vi "RTI Connext DDS Secure Shapes Reader.vi"() -> ()   [LabVIEW 2012]
doc: "Shows how to subscribe to an existing RTI Connext DDS application: RTI Shapes Demo. It was created using the Tutorial of the Getting Started Guide (<LabVIEW folder>/help/RTI DDS Toolkit for LabVIEW/RTI_DDS_Toolkit_for_LabVIEW_GettingStarted.pdf)."
uses:
  RTI/GIT_HEAD/connextdds/lvdds.1.0/srcLV/lvdds.1.0_package/Examples/ShapesDemo/RTI Connext DDS Shape Type.ctl
  RTI/GIT_HEAD/connextdds/lvdds.1.0/srcLV/lvdds.1.0_package/Types/DDS Sample Info.ctl
  RTI/GIT_HEAD/connextdds/lvdds.1.0/srcLV/lvdds.1.0_package/Types/RTI DDS Advanced Reader Configuration.ctl
  RTI/GIT_HEAD/connextdds/lvdds.1.0/srcLV/lvdds.1.0_package/Types/RTI DDS Security Settings.ctl
  RTI/GIT_HEAD/connextdds/lvdds.1.0/srcLV/lvdds.1.0_package/Types/RTI DDS Basic Security Settings.ctl
  RTI/GIT_HEAD/connextdds/lvdds.1.0/srcLV/lvdds.1.0_package/Types/RTI DDS Advanced Security Settings.ctl
  RTI/GIT_HEAD/connextdds/lvdds.1.0/srcLV/lvdds.1.0_package/Library/LVDDS_library.lvlib
  RTI/GIT_HEAD/connextdds/lvdds.1.0/lib/rtilvdds.dll
panel:
  in  "Domain Id":u32
  in  "Topic Name":string(combo)="Square"
  in  "error in (no error)":errorcluster
  in  "Advanced Reader Configuration":T1
  in  "Enter a shape 'color' to see the square moving in 'XY Graph' and its size in 'shapesize'":string
  out "Sample Info":T2
  out "Return value 2":i32
  out "DDS Data":string[][](table)
  in  "Enable DDS":bool
  in  "ShapeType 2":T3
  out "XY Graph":cluster{"Y":dbl[], "Y":dbl[]}[](graph)
  out "shapesize":i32(slide) scale=0.0..100.0
  in  "Query condition":string
  in  "Stop":bool
  out "Shape 2":T4
  out "Return value":i32
  # "This Example will show Security capabilities using RTI Shapes Demo example. \n\nRTI Shapes Demo is a sample application that demonstrates DDS concepts. It can publish and subscribe to data of type “ShapeType”, which consists of color, x and y coordinates, and a shapesize.  You can use this example to subscribe to Secure Shapes data using  RTI Connext. Run RTI Shapes Demo 5.2.4 or above or the Secure Shapes Writer.vi to publish entities. Start this Shapes Reader example VI, and click on 'DDS  Stopped' below to start reading. Published Shapes data will be displayed. \nIf you want to see one of the shapes moving in the XY Graph, enter its color (in capital letters) in the box below."
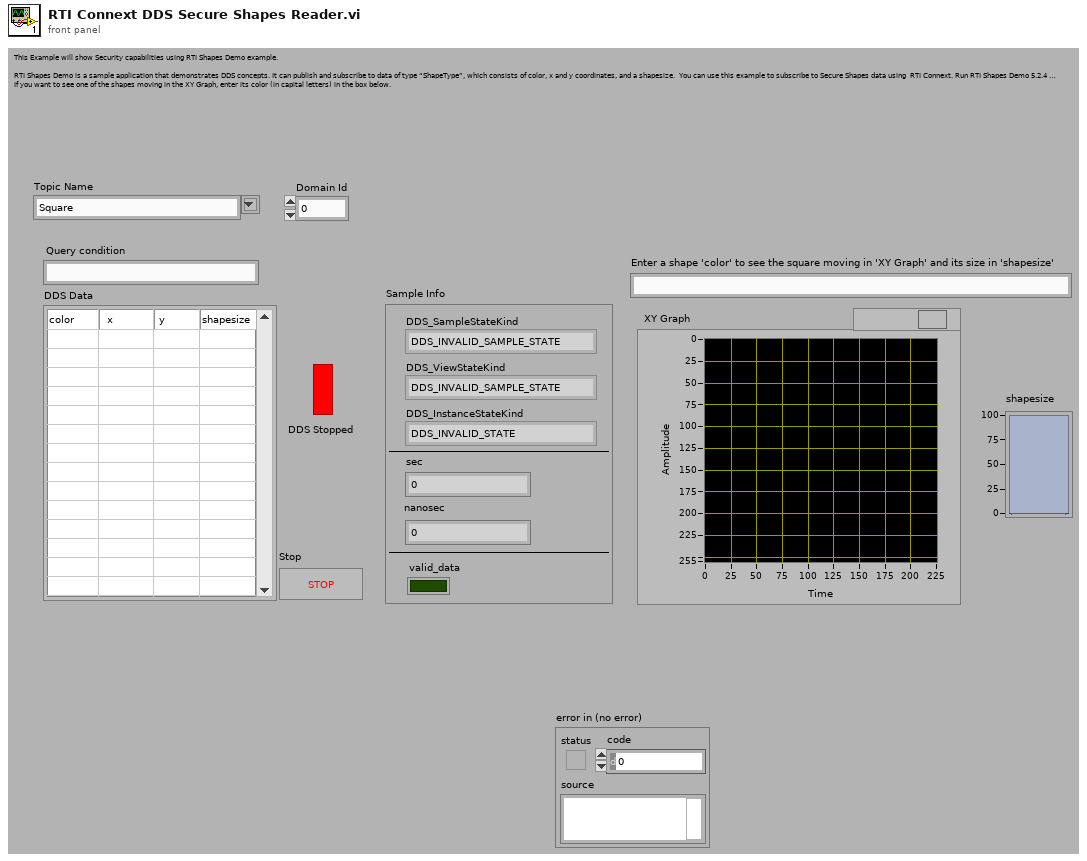
[diagram p1: front panel]
types:
  T1 = typedef "LVDDS_library.lvlib/RTI DDS Advanced Reader Configuration.ctl" = cluster{"typeName":string, "keyName":string, "domainParticipantQoSProfile":string, "dataReaderQoSProfile":string, "forceNewDomainParticipant?":bool, "forceArrayMapping?":bool, "forceExclusiveReader?":bool, "forceRead? (only ExclusiveReader)":bool, "forceUnboundedString?":bool}
  T2 = typedef "LVDDS_library.lvlib/DDS Sample Info.ctl" = cluster{"DDS_SampleStateKind":enum32{"DDS_INVALID_SAMPLE_STATE", "DDS_READ_SAMPLE_STATE", "DDS_NOT_READ_SAMPLE_STATE"}, "DDS_ViewStateKind":enum32{"DDS_INVALID_SAMPLE_STATE", "DDS_NEW_VIEW_STATE", "DDS_NOT_NEW_VIEW_STATE"}, "DDS_InstanceStateKind":enum32{"DDS_INVALID_STATE", "DDS_ALIVE_INSTANCE_STATE", "DDS_NOT_ALIVE_DISPOSED_INSTANCE_STATE", "", "DDS_NOT_ALIVE_NO_WRITERS_INSTANCE_STATE"}, "sec":i32, "nanosec":u32, "valid_data":bool}
  T3 = cluster{"Color":string, "x":i32, "y":i32, "shapesize":i32}
  T4 = typedef "RTI Connext DDS Shape Type.ctl" = cluster{"color":string, "x":i32, "y":i32, "shapesize":i32}
  T5 = typedef "LVDDS_library.lvlib/RTI DDS Security Settings.ctl" = cluster{"Basic Security Settings":T6, "Advanced Security Settings":T7}
  T6 = typedef "LVDDS_library.lvlib/RTI DDS Basic Security Settings.ctl" = cluster{"Identity Certificate Authority (CA)":path, "Identity Certificate (Signed by Identity CA)":path, "Private Key":path, "Permissions Certificate Authority (CA)":path, "Governance Document (Signed by Permissions CA)":path, "Permissions Document (Signed by Permissions CA)":path}
  T7 = typedef "LVDDS_library.lvlib/RTI DDS Advanced Security Settings.ctl" = cluster{"Shared Secret Algorithm":string, "Encryption Algorithm":string, "Certificate Revocation List":path}
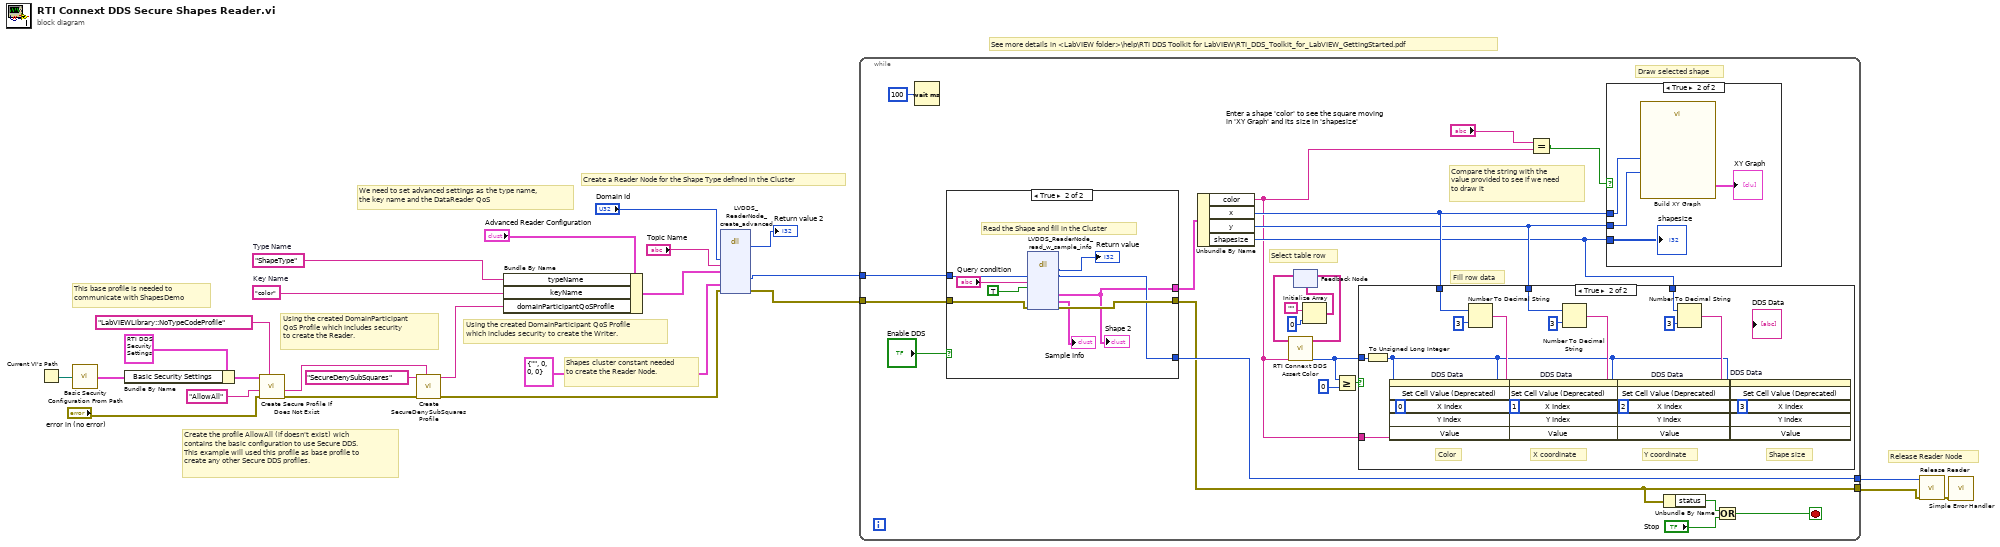
[diagram p0: block diagram]
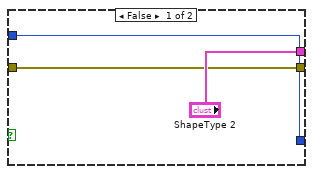
[diagram p3: hidden frame]
diagram:
  w15 = "color"  # Key Name
  w14 = "ShapeType"  # Type Name
  # "Using the created DomainParticipant \nQoS Profile which includes security \nto create the Reader."
  # "Create the profile AllowAll (if doesn't exist) wich \ncontains the basic configuration to use Secure DDS.\nThis example will used this profile as base profile to \ncreate any other Secure DDS profiles."
  # "This base profile is needed to \ncommunicate with ShapesDemo"
  # "Using the created DomainParticipant QoS Profile\nwhich includes security to create the Writer."
  # "See more details in <LabVIEW folder>\\help\\RTI DDS Toolkit for LabVIEW\\RTI_DDS_Toolkit_for_LabVIEW_GettingStarted.pdf"
  # "We need to set advanced settings as the type name,\nthe key name and the DataReader QoS"
  # "Release Reader Node"
  # "Shapes cluster constant needed to create the Reader Node."
  # "Create a Reader Node for the Shape Type defined in the Cluster"
  n1 = Current VI's Path() -> (path=w7:path)
  n2 = call "Basic Security Configuration From Path.vi"("Current Path"=w7) -> ("Basic Security Settings"=w9:T6)
  n3 = Bundle By Name(cluster=T5 {"Basic Security Settings"={"Identity Certificate Authority (CA)"=path "", "Identity Certificate (Signed by Identity CA)"=path "", "Private Key"=path "", "Permissions Certificate Authority (CA)"=path "", "Governance Document (Signed by Permissions CA)"=path "", "Permissions Document (Signed by Permissions CA)"=path ""}, "Advanced Security Settings"={"Shared Secret Algorithm"="ecdsa-ecdh", "Encryption Algorithm"="aes-128-gcm", "Certificate Revocation List"=path ""}} ("Security Settings"), "Basic Security Settings"=w9) -> (w8:T5)
  n4 = call "Create Secure Profile If Does Not Exist.vi"("Base Profile"="LabVIEWLibrary::NoTypeCodeProfile", "error in (no error)"="error in (no error)", "New Profile Name"="AllowAll", "Security Settings"=w8) -> ("error out"=w5:errorcluster, "New Profile Name Output"=w4:string)  [unwired: 6 in]
  n5 = call "Create SecureDenySubSquares Profile.vi"("DomainParticipant Base Profile Name"=w4, "error in (no error)"=w5, "New Custom Secure Profile Name"="SecureDenySubSquares") -> ("error out"=w2:errorcluster, "Custom Secure Profile Name Output"=w1:string)  [unwired: 7 in]
  n6 = Bundle By Name(cluster="Advanced Reader Configuration", "typeName"=w14, "keyName"=w15, "domainParticipantQoSProfile"=w1) -> (w13:T1)
  n7 = dll-call lib="D:/RTI/GIT_HEAD/connextdds/lvdds.1.0/lib/rtilvdds.*" fn="LVDDS_ReaderNode_create_advanced"("domain id"="Domain Id", "topic name"="Topic Name", "advanced reader configuration"=w13, "data type"=T4 {"color"="", "x"=0, "y"=0, "shapesize"=0} ("Shape 3"), "error"=w2) -> ("return type"=→"Return value 2":i32, "ref num"=w21:u64, "error"=w20:errorcluster)  [unwired: 10 in, 2 out]
  n8 = while {
    tunnel: w21 -> [w35]
    tunnel: [w40] -> w25
    tunnel: w20 -> [w34]
    tunnel: [w31] -> w24
    stop <- w32 stop-if-true
    # "Compare the string with the\nvalue provided to see if we need\nto draw it"
    # "Select table row"
    # "Draw selected shape"
    # "Fill row data"
    n9 = Wait (ms)(milliseconds to wait=u32 100) -> ()  [unwired: 1 out]
    n10 = case shown="True" "Enable DDS" {
      tunnel: ["ShapeType 2" w69] -> w47
      tunnel: w35 -> [w67 w77]
      tunnel: [w67 w73] -> w40
      tunnel: w34 -> [w66 w75]
      tunnel: [w66 w74] -> w31
      frame False {
      }
      frame True {
        # "Read the Shape and fill in the Cluster"
        n11 = dll-call lib="D:/RTI/GIT_HEAD/connextdds/lvdds.1.0/lib/rtilvdds.*" fn="LVDDS_ReaderNode_read_w_sample_info"("Ref Num"=w77, "Query Condition"="Query condition", "Only new?"=TRUE ("Read All Samples"), "Error"=w75) -> ("return type"=→"Return value":i32, "Ref Num"=w73:u64, "Shape"=w69:T4, "Sample Info"=→"Sample Info":T2, "Error"=w74:errorcluster)  [unwired: 7 in, 2 out]
        "Shape 2" <- w69
      }
    }
    n12 = Unbundle By Name(w47) -> ("color"=w26:string, "x"=w49:i32, "y"=w48:i32, "shapesize"=w43:i32)
    n13 = Initialize Array("", 0 ("dimension size")) -> (w44:string[])
    n14 = feedback #1(w44) -> (w37:string[])
    n15 = call "RTI Connext DDS Assert Color.vi"("Color"=w26, "Input Array"=w37) -> ("Position"=w36:i32, "Output Array"=w38:string[])  [unwired: 8 in]
    n16 = feedback-in #1(w38) -> ()
    n17 = Greater Or Equal?(x=w36, y=0) -> (x >= y?=w42:bool)
    n18 = case shown="True" w42 {
      tunnel: w49 -> [_ w55]
      tunnel: w48 -> [_ w54]
      tunnel: w36 -> [_ w51]
      tunnel: w26 -> [_ w53]
      tunnel: w43 -> [_ w52]
      frame False {
      }
      frame True {
        # "Shape size"
        # "Y coordinate"
        # "X coordinate"
        # "Color"
        n19 = To Unsigned Long Integer(number=w51) -> (unsigned 32bit integer=w50:u32)
        n20 = invoke on="DDS Data" class="Tbl (strict)" method="Set Cell Value (Deprecated)"("X Index"=u32 0, "Y Index"=w50, "Value"=w53) -> ()  [unwired: 3 in, 6 out]
        n21 = Number To Decimal String(number=w55, width (-)=3) -> (decimal integer string=w60:string)
        n22 = invoke on="DDS Data" class="Tbl (strict)" method="Set Cell Value (Deprecated)"("X Index"=u32 1, "Y Index"=w50, "Value"=w60) -> ()  [unwired: 3 in, 6 out]
        n23 = Number To Decimal String(number=w54, width (-)=3) -> (decimal integer string=w56:string)
        n24 = invoke on="DDS Data" class="Tbl (strict)" method="Set Cell Value (Deprecated)"("X Index"=u32 2, "Y Index"=w50, "Value"=w56) -> ()  [unwired: 3 in, 6 out]
        n25 = Number To Decimal String(number=w52, width (-)=3) -> (decimal integer string=w58:string)
        n26 = invoke on="DDS Data" class="Tbl (strict)" method="Set Cell Value (Deprecated)"("X Index"=u32 3, "Y Index"=w50, "Value"=w58) -> ()  [unwired: 3 in, 6 out]
      }
    }
    n27 = Equal?(x="Enter a shape 'color' to see the square moving in 'XY Graph' and its size in 'shapesize'", y=w26) -> (x = y?=w28:bool)
    n28 = case shown="True" w28 {
      tunnel: w49 -> [_ w78]
      tunnel: w48 -> [_ w80]
      tunnel: w43 -> [_ w79]
      frame False {
      }
      frame True {
        n29 = call "Build XY Graph"("Y Input"=w80, "X Input"=w78) -> ("XY Graph"=→"XY Graph":cluster{"Y":dbl[], "Y":dbl[]}[])  [unwired: 3 in, 6 out]
        "shapesize" <- w79
      }
    }
    n30 = Unbundle By Name(w31) -> ("status"=w29:bool)
    n31 = Or(x=w29, y="Stop") -> (x .or. y?=w32:bool)
  }
  n32 = call "Release Reader.vi"("error in"=w24, "ref num"=w25) -> ("error out"=w23:errorcluster)  [unwired: 9 in]
  n33 = call <vilib>:"Simple Error Handler.vi"("error in (no error)"=w23) -> ()  [unwired: 4 in, 5 out]
